vi "ReadWriteLoopCase6.vi"() -> ()   [LabVIEW 2019]
uses:
  <vilib>/Platform/TimedLoop/XDataNode/timing_clust.ctl
  <vilib>/Platform/TimedLoop/XDataNode/nitl_modes.ctl
  <vilib>/Platform/TimedLoop/XDataNode/wakeup.ctl
  <vilib>/DAQmx/read.llb/DAQmx Read (Analog DBL 1Chan 1Samp).vi
  <vilib>/DAQmx/write.llb/DAQmx Write (Analog DBL 1Chan 1Samp).vi
  <vilib>/DAQmx/create/channels.llb/DAQmx Create Channel (AI-Voltage-Basic).vi
  <vilib>/DAQmx/create/channels.llb/DAQmx Create Channel (AO-Voltage-Basic).vi
  <vilib>/DAQmx/configure/timing.llb/DAQmx Timing (Sample Clock).vi
  <vilib>/DAQmx/create/timing.llb/DAQmx Create Timing Source (Signal From Task).vi
  <vilib>/DAQmx/miscellaneous.llb/DAQmx Fill In Error Info.vi
  <vilib>/platform/TimedLoop/XDataNode/XDataNode.xnode
  <resource>/objmgr/daqmx.rc
  <vilib>/Platform/TimedLoop/XDataNode/XDNodeRunTimeDep.lvlib
panel:
  out "Finished Late? [i-1]":bool
  out "Actual End [i-1]":i64
  out "Expected End [i-1]":i64
  in  "stop":bool
  out "1/x":dbl
  out "Specified Write Rate":dbl
  out "Specified Sampling Rate":dbl
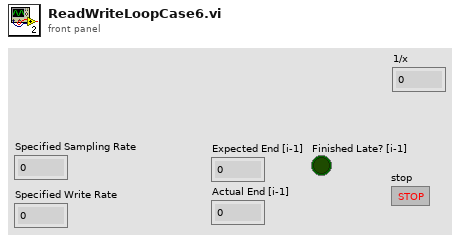
[diagram p1: front panel]
types:
  T1 = typedef "XDNodeRunTimeDep.lvlib/timing_clust.ctl" = cluster{"Expected End [f-1]":u64, "Actual End [f-1]":u64, "Finished Late? [f-1]":bool, "Expected End [i-1]":u64, "Actual End [i-1]":u64, "Finished Late? [i-1]":bool, "Expected Start [i]":u64, "Actual Start [i]":u64, "Expected Start [f]":u64, "Actual Start [f]":u64, "Source Name":string, "Structure Name":string, "Period":i64, "Deadline":i64, "Offset":i64, "Start":i64, "Priority":i32, "Timeout":i32, "Mode":T2, "Wakeup Reason":T3, "Error":errorcluster, "Source Type":string, "Secondary Source Type":string, "Global End Time":u64, "Global Start Time":u64, "Frame Duration":u64, "Iteration Duration":u64, "Assigned CPU":i32, "I/O Scan Engine Mode":u32}
  T2 = typedef "XDNodeRunTimeDep.lvlib/nitl_modes.ctl" = enum32{"No Change", "Process missed periods, maintain original phase", "Discard missed periods, maintain original phase", "Process missed periods, ignore original phase", "Discard missed periods, ignore original phase"}
  T3 = typedef "XDNodeRunTimeDep.lvlib/wakeup.ctl" = enum32{"Normal", "Aborted", "Asynchronous wakeup", "Timing source error", "Timed loop error", "Timeout"}
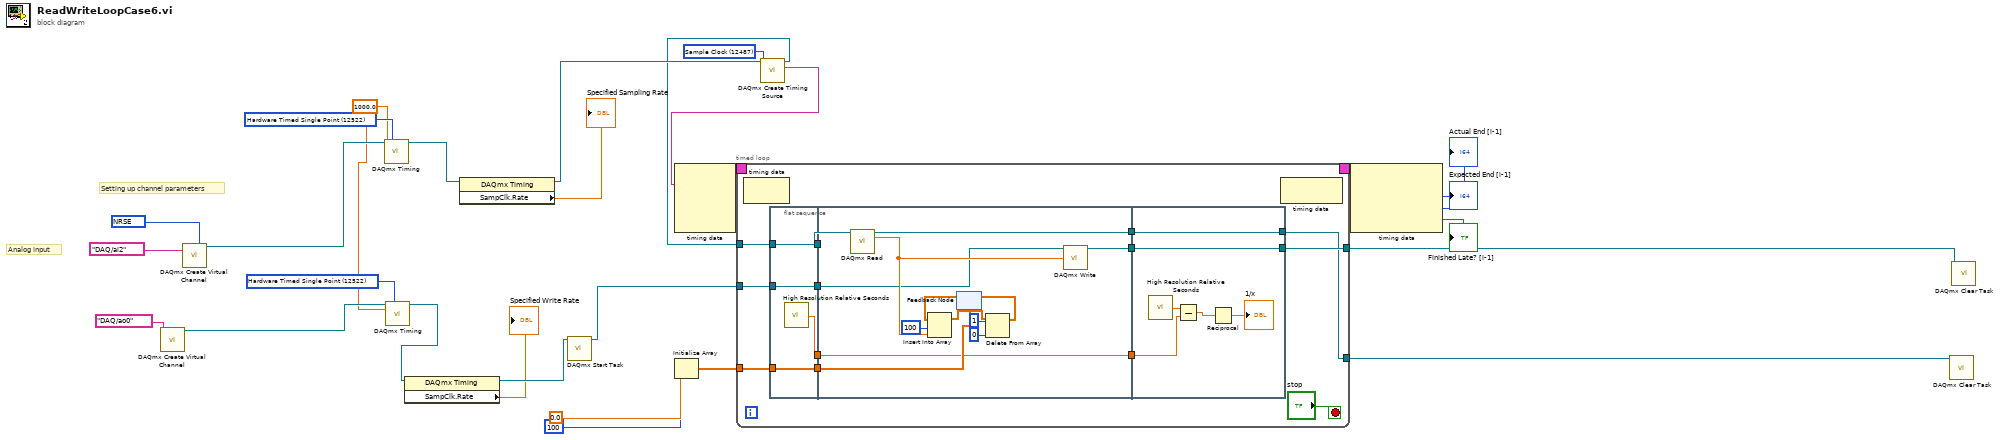
[diagram p0: block diagram]
diagram:
  w2 = 12522 items=["Finite Samples"=10178, "Continuous Samples"=10123, "Hardware Timed Single Point"=12522] ("sample mode")
  w4 = 12487 items=["Sample Complete Event"=12530, "Counter Output Event"=12494, "Change Detection Event"=12511, "Sample Clock"=12487] ("signal")
  w7 = 1000.0 ("rate")
  w10 = 12522 items=["Finite Samples"=10178, "Continuous Samples"=10123, "Hardware Timed Single Point"=12522] ("sample mode")
  w26 = 10078 items=["Default"=-1, "RSE"=10083, "NRSE"=10078, "Differential"=10106, "Pseudodifferential"=12529] ("input terminal configuration")
  # "Analog input"
  # "Setting up channel parameters"
  n1 = call-poly <vilib>:"DAQmx Create Virtual Channel.vi"("physical channels"=tag "DAQ/ao0") -> ("task out"=w9:refnum<k21>)  [unwired: 13 in, 1 out]
  n2 = call-poly <vilib>:"DAQmx Create Virtual Channel.vi"("input terminal configuration"=w26, "physical channels"=tag "DAQ/ai2") -> ("task out"=w11:refnum<k21>)  [unwired: 12 in, 1 out]
  n3 = call-poly <vilib>:"DAQmx Timing.vi"("task/channels in"=w11, "sample mode"=w10, "rate"=w7) -> ("task out"=w6:refnum<k21>)  [unwired: 11 in, 1 out]
  n4 = call-poly <vilib>:"DAQmx Timing.vi"("task/channels in"=w9, "sample mode"=w2, "rate"=w7) -> ("task out"=w8:refnum<k21>)  [unwired: 11 in, 1 out]
  n5 = property class="DAQmx Timing"(reference=w8) -> (reference out=w23:refnum<k21>, "SampClk.Rate"=→"Specified Write Rate":dbl)  [unwired: 1 in, 1 out]
  n6 = property class="DAQmx Timing"(reference=w6) -> (reference out=w5:refnum<k21>, "SampClk.Rate"=→"Specified Sampling Rate":dbl)  [unwired: 1 in, 1 out]
  n7 = call <vilib>:"DAQmx Start Task.vi"("task/channels in"=w23) -> ("task out"=w12:refnum<k21>)  [unwired: 13 in, 1 out]
  n8 = Initialize Array(0.0 ("element"), 100 ("dimension size")) -> (w15:dbl[])
  n9 = call-poly <vilib>:"DAQmx Create Timing Source.vi"("task/channels in"=w5, "signal"=w4) -> ("task out"=w1:refnum<k21>, "timing source out"=w3:string)  [unwired: 11 in, 1 out]
  n10 = node-c288(w3) -> (w28:T1)  [unwired: 3 in]
  n11 = timed-loop {
    timing: w28 -> [_]
    timing-out: [_] -> w27
    tunnel: w1 -> [w41]
    tunnel: w15 -> [w40]
    tunnel: [w38] -> w14
    tunnel: [w37] -> w13
    tunnel: w12 -> [w36]
    stop <- "stop" stop-if-true
    n12 = node-c288() -> ()  [unwired: 1 in, 1 out]
    n13 = flat-sequence {
      tunnel: w36 -> [w43]
      tunnel: w40 -> [w44]
      tunnel: w41 -> [w45]
      tunnel: [w45] -> w35
      tunnel: [w44] -> w34
      tunnel: [w43] -> w33
      tunnel: [w42] -> w30
      tunnel: w35 -> [w58]
      tunnel: w34 -> [w50]
      tunnel: w33 -> [w47]
      tunnel: [w49] -> w32
      tunnel: [w48] -> w31
      tunnel: w30 -> [w46]
      tunnel: [w46] -> w29
      tunnel: [w63] -> w37
      tunnel: [w64] -> w38
      tunnel: w32 -> [w64]
      tunnel: w31 -> [w63]
      tunnel: w29 -> [w61]
      frame #0 {
        n14 = call <vilib>:"High Resolution Relative Seconds.vi"() -> ("relative seconds"=w42:dbl)
      }
      frame #1 {
        n15 = call-poly <vilib>:"DAQmx Read.vi"("task/channels in"=w58) -> ("task out"=w48:refnum<k21>, "data"=w57:dbl)  [unwired: 12 in, 1 out]
        n16 = feedback #1(w50) -> (w51:dbl[])
        n17 = Insert Into Array(array=w51, index=100, new element=w57) -> (w53:dbl[])
        n18 = Delete From Array(array=w53, length=1, index=0) -> (array with subset deleted=w52:dbl[])  [unwired: 1 out]
        n19 = feedback-in #1(w52) -> ()
        n20 = call-poly <vilib>:"DAQmx Write.vi"("task/channels in"=w47, "data"=w57) -> ("task out"=w49:refnum<k21>)  [unwired: 11 in, 2 out]
      }
      frame #2 {
        n21 = call <vilib>:"High Resolution Relative Seconds.vi"() -> ("relative seconds"=w62:dbl)
        n22 = Subtract(x=w62, y=w61) -> (x-y=w60:dbl)
        n23 = Reciprocal(x=w60) -> (1/x=→"1/x":dbl)
      }
    }
    n24 = node-c288() -> ()  [unwired: 1 in, 1 out]
  }
  n25 = node-c288(w27) -> (→"Expected End [i-1]":i64, →"Actual End [i-1]":i64, →"Finished Late? [i-1]":bool)  [unwired: 1 out]
  n26 = call <vilib>:"DAQmx Clear Task.vi"("task in"=w13) -> ()  [unwired: 14 in, 1 out]
  n27 = call <vilib>:"DAQmx Clear Task.vi"("task in"=w14) -> ()  [unwired: 14 in, 1 out]
